vi "Enqueue (Array).vi"(6 "Priority Message? Array":bool[](array[boolean]), 7 "timeout in ms (-1)":i32=-1, 8 "error in (no error)":errorcluster, 9 "Message Data Array":variant[](array[variant]), 10 "States":T2[](array[typedef]), 11 "Message Queue":T1) -> (0 "error out":errorcluster, 3 "Message Queue dub":T1)   [LabVIEW 2019, in "Test.lvlib"]
doc: "For a regular message, enqueue the message. For a priority message, enqueue it at the front of the queue."
uses:
  Test.lvlib
  State Name.ctl
  Support/Shared/TypeDefs/Message Queue Ref.ctl
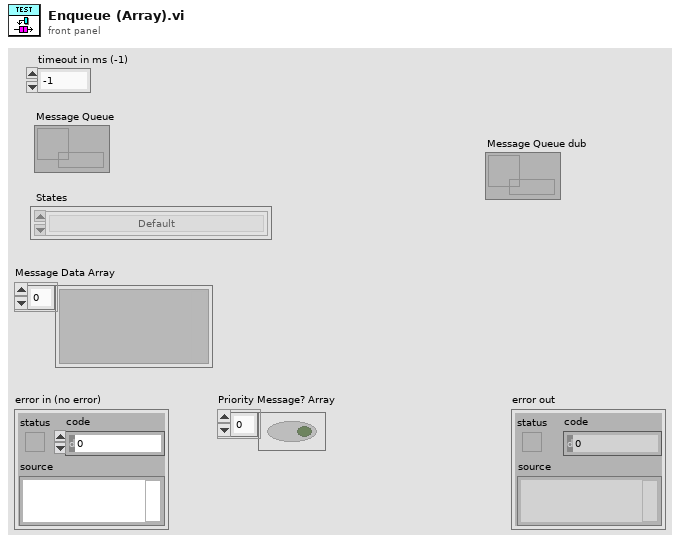
[diagram p1: front panel]
types:
  T1 = typedef "Message Queue Ref.ctl" = refnum<queue>
  T2 = typedef "Test.lvlib/State Name.ctl" = enum16{"Default", "Initialize", "Re-Initialize", "Initialize Data", "Initialize Panel", "[Event Structure] Update Data", "Error", "Exit"}
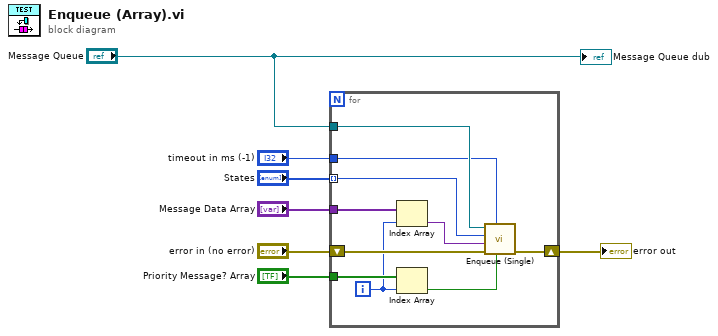
[diagram p0: block diagram]
diagram:
  n1 = for {
    tunnel: "Message Data Array" -> [w13]
    tunnel: "Priority Message? Array" -> [w10]
    tunnel: "Message Queue" -> [w15]
    shift-right: [w14] -> w4
    shift-left: "error in (no error)" -> [w17]
    tunnel: "States" -> [w16] mode=indexing
    tunnel: "timeout in ms (-1)" -> [w11]
    i -> [w9]
    n2 = Index Array(array=w13, index=w9) -> (element=w12:variant)
    n3 = Index Array(array=w10, index=w9) -> (element=w8:bool)
    n4 = call "Enqueue (Single).vi"("Priority Message? Array"=w8, "timeout in ms (-1)"=w11, "error in (no error)"=w17, "Message Data Array"=w12, "States"=w16, "Message Queue"=w15) -> ("error out"=w14:errorcluster)  [unwired: 4 in, 1 out]
  }
  "error out" <- w4
  "Message Queue dub" <- "Message Queue"
